vi "Scale.vi"   [LabVIEW 2020, in "NI ECAT Remote IO.lvlib"]
doc: "Manages conversion between raw data and scaled data."
uses:
  <vilib>/indcomecat/Remote IO/NI ECAT Remote IO.lvlib
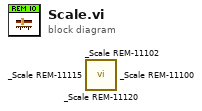
[diagram p0: block diagram]
diagram:
  n1 = call <vilib>:"_Scale REM-11120.vi"() -> ()  [unwired: 10 in, 2 out]
  n2 = call <vilib>:"_Scale REM-11102.vi"() -> ()  [unwired: 10 in, 2 out]
  n3 = call <vilib>:"_Scale REM-11115.vi"() -> ()  [unwired: 10 in, 2 out]
  n4 = call <vilib>:"_Scale REM-11100.vi"() -> ()  [unwired: 10 in, 2 out]
